vi "XYZTheta Go.vi"(8 "error in (no error)":errorcluster, 10 "XYZTheta In":dbl[](array[numeric]), 11 "Gantry 2":refnum<k24>) -> (0 "error out":errorcluster, 2 "XYZTheta Out":dbl[](array[numeric]), 3 "Gantry 3":refnum<k24>)   [LabVIEW 2020, in "Motion.lvclass"]
uses:
  Motion.lvclass
  C:/Program Files (x86)/Aerotech/A3200/LabVIEW/2010/Bin/Aerotech.A3200.dll
  Program Files (x86)/Aerotech/A3200/LabVIEW/2010/Bin/Aerotech.A3200.dll
  A3200/A3200.lvclass
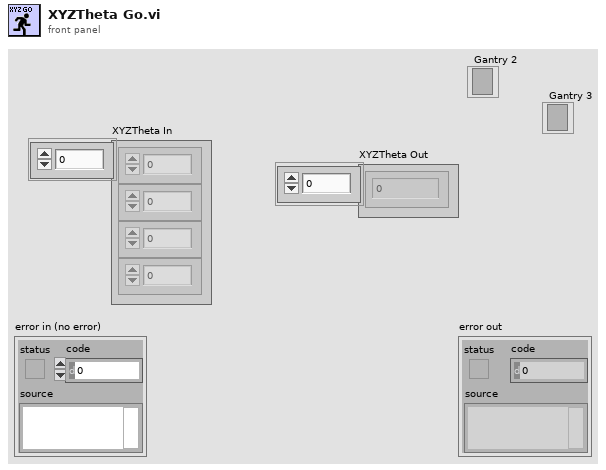
[diagram p1: front panel]
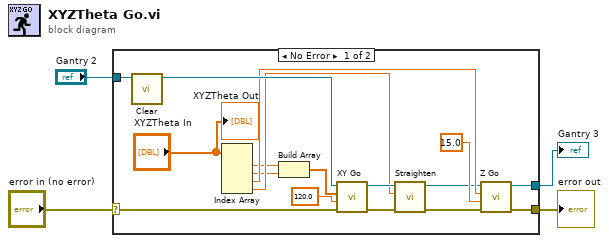
[diagram p0: block diagram]
diagram:
  n1 = case shown="No Error" "error in (no error)" {
    selector: "error in (no error)" -> [w8 w23]
    tunnel: [w5 w23] -> w3
    tunnel: "Gantry 2" -> [w20 w22]
    tunnel: [w12 w22] -> w1
    frame No Error {
      n2 = call "Clear.vi"("Gantry 2"=w20) -> ("Gantry 3"=w19:refnum<k24>)  [unwired: 9 in, 1 out]
      n3 = Index Array(array="XYZTheta In") -> (element #1=w10:dbl, element #2=w9:dbl, element #3=w15:dbl, element #4=w16:dbl)  [unwired: 4 in]
      n4 = Build Array(w10, w9) -> (w11:dbl[])
      n5 = call "XY Go.vi"("error in (no error)"=w8, "Speed"=120.0, "XY"=w11, "Gantry 2"=w19) -> ("error out"=w7:errorcluster, "Gantry 3"=w17:refnum<k24>)  [unwired: 6 in]
      n6 = call "Straighten.vi"("error in (no error)"=w7, "Angle (rad)"=w16, "Gantry 2"=w17) -> ("error out"=w6:errorcluster, "Gantry 3"=w13:refnum<k24>)  [unwired: 7 in]
      n7 = call "Z Go.vi"("error in (no error)"=w6, "Speed"=15.0, "Position"=w15, "Gantry 2"=w13) -> ("error out"=w5:errorcluster, "Gantry 3"=w12:refnum<k24>)  [unwired: 6 in]
      "XYZTheta Out" <- "XYZTheta In"
    }
    frame Error {
    }
  }
  "error out" <- w3
  "Gantry 3" <- w1
